vi "GetMessage.vi"(11 "ExampleClass in":refnum<class "ExampleClass.lvclass">) -> (2 "Message":string, 3 "ExampleClass out":refnum<class "ExampleClass.lvclass">)   [LabVIEW 2012, in "ExampleClass.lvclass"]
uses:
  ExampleClass.lvclass
  ExampleClass.lvclass/ExampleClass.ctl
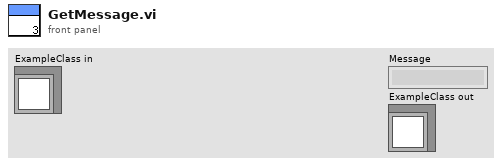
[diagram p1: front panel]
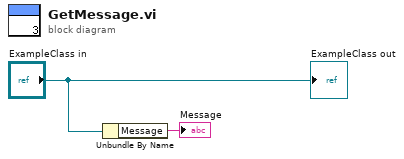
[diagram p0: block diagram]
diagram:
  n1 = Unbundle By Name("ExampleClass in") -> ("Message"=→"Message":string)
  "ExampleClass out" <- "ExampleClass in"
